vi "引用测试.vi"() -> ()   [LabVIEW 2019, in "test.lvlib"]
uses:
  SubVI/335 state.ctl
  SubVI/test.lvlib
panel:
  out "下拉列表 3":T1=2 items=["Unknow", "Stable", "Following Warm", "Following Cold", "Unfollowing"]
  out "下拉列表 2":T1=2 items=["Unknow", "Stable", "Following Warm", "Following Cold", "Unfollowing"]
  in  "下拉列表":T1=2 items=["Unknow", "Stable", "Following Warm", "Following Cold", "Unfollowing"]
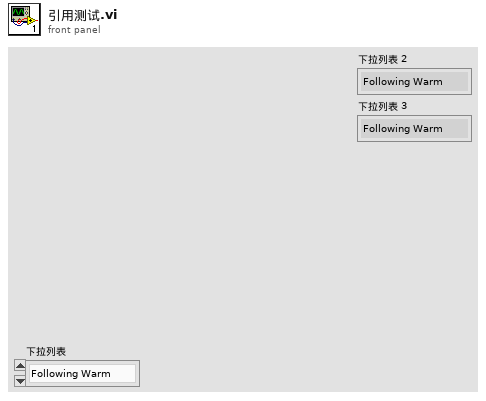
[diagram p1: front panel]
types:
  T1 = typedef "335 state.ctl" = u16
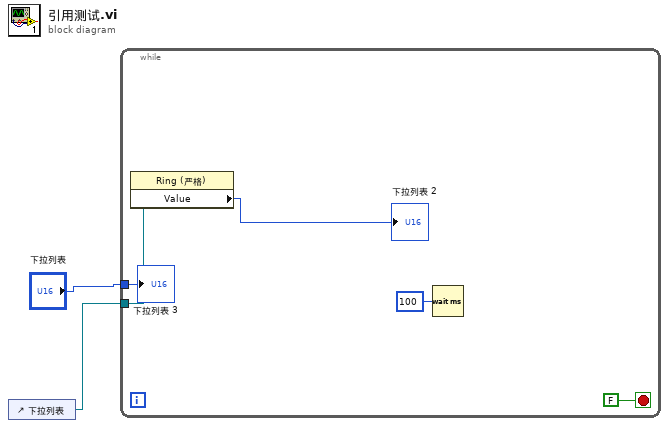
[diagram p0: block diagram]
diagram:
  n1 = control-ref of="下拉列表"() -> (w2:refnum<vi>)
  n2 = while {
    tunnel: w2 -> [w7]
    tunnel: "下拉列表" -> [w3]
    stop <- FALSE stop-if-true
    n3 = property class="Ring (严格)"(reference=w7) -> ("Value"=→"下拉列表 2":T1)  [unwired: 1 in, 2 out]
    n4 = Wait (ms)(milliseconds to wait=u32 100 ("等待时间（毫秒）")) -> ()  [unwired: 1 out]
    "下拉列表 3" <- w3
  }
